vi "TestSquare.vi"(11 "error in (no error)":errorcluster) -> (15 "error out":errorcluster)   [LabVIEW 2016, in "SimpleCalculatorTests.lvlib"]
doc: "Performs square test"
uses:
  SimpleCalculatorTests.lvlib
  APIs/Stimulus/ControlValue/SetValueAuto.vi
  APIs/Get/GetVI/GetVIByName.vi
  APIs/Assert/AssertControlValue/AlmostEqual.vi
  APIs/Stimulus/VI/CloseVI.vi
  Drona.lvlib
  <vilib>/addons/_JKI Toolkits/Caraya/classes/Test/Test.lvclass
  APIs/Stimulus/ControlValue/ControlValue.lvlib
  APIs/Assert/AssertControlValue/AssertControlValue.lvlib
  APIs/Get/GetVI/GetVI.lvlib
  APIs/Stimulus/VI/VI.lvlib
panel:
  # "Drona Test Square"
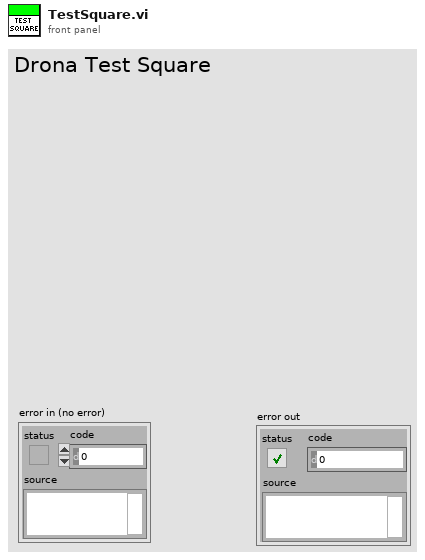
[diagram p1: front panel]
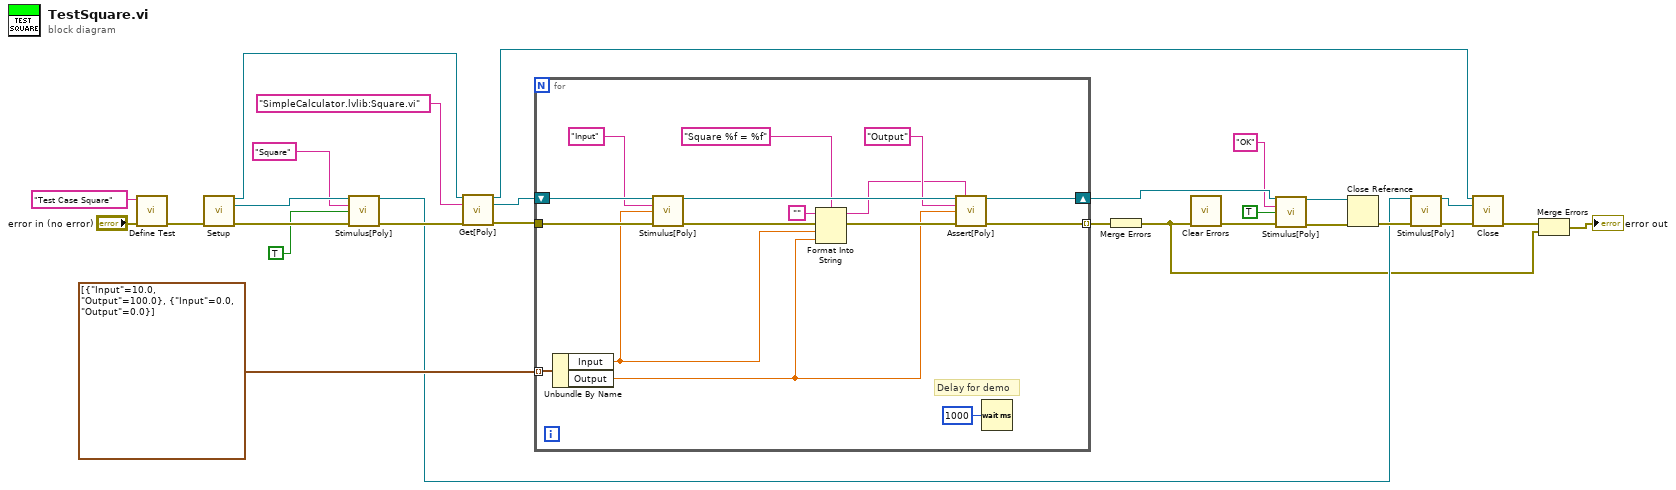
[diagram p0: block diagram]
diagram:
  n1 = call <vilib>:"Define Test.vi"("error in (no error)"="error in (no error)", "Label (VI Title)"="Test Case Square") -> ("error out"=w28:errorcluster)  [unwired: 9 in]
  n2 = call "Setup.vi"("error in"=w28) -> ("Application Ref"=w17:refnum<vi>, "VI Reference Out"=w24:refnum<vi>, "error out"=w25:errorcluster)  [unwired: 12 in]
  n3 = call-poly "Stimulus[Poly].vi"("VI Reference In"=w24, "Control Path"="Square", "Value (Signaling)"=TRUE, "error in"=w25) -> ("VI Reference Out"=w7:refnum<vi>, "error out"=w21:errorcluster)  [unwired: 10 in]
  n4 = call-poly "Get[Poly].vi"("Application Ref in"=w17, "VI Name"="SimpleCalculator.lvlib:Square.vi" ("Control Path"), "error in (no error)"=w21) -> ("Application Ref out"=w16:refnum<vi>, "VI Reference"=w18:refnum<vi>, "error out"=w19:errorcluster)  [unwired: 10 in]
  n5 = for {
    shift-right: [w38] -> w15
    shift-left: w18 -> [w44]
    tunnel: cluster{"Input":dbl, "Output":dbl}[] [{"Input"=10.0, "Output"=100.0}, {"Input"=0.0, "Output"=0.0}] -> [w36] mode=indexing
    tunnel: w19 -> [w43]
    tunnel: [w39] -> w14 mode=indexing
    # "Delay for demo"
    n6 = Unbundle By Name(w36) -> ("Input"=w33:dbl, "Output"=w32:dbl)
    n7 = call-poly "Stimulus[Poly].vi"("VI Reference In"=w44, "Control Path"="Input", "Value (Signaling)"=w33, "error in"=w43) -> ("VI Reference Out"=w40:refnum<vi>, "error out"=w41:errorcluster)  [unwired: 10 in]
    n8 = Format Into String(format string="Square %f = %f", initial string="", error in=w41, w33, w32) -> (resulting string=w31:string, error out=w35:errorcluster)
    n9 = call-poly "Assert[Poly].vi"("VI Reference In"=w40, "Test Label"=w31, "Control Path"="Output", "Control Value"=w32, "Error In"=w35) -> ("VI Reference Out"=w38:refnum<vi>, "Error Out"=w39:errorcluster)  [unwired: 9 in]
    n10 = Wait (ms)(milliseconds to wait=u32 1000) -> ()  [unwired: 1 out]
  }
  n11 = Merge Errors(w14) -> (w2:errorcluster)
  n12 = call <vilib>:"Clear Errors.vi"("error in (no error)"=w2) -> ("error out"=w9:errorcluster)  [unwired: 5 in, 1 out]
  n13 = call-poly "Stimulus[Poly].vi"("VI Reference In"=w15, "Control Path"="OK", "Value (Signaling)"=TRUE, "error in"=w9) -> ("VI Reference Out"=w12:refnum<vi>, "error out"=w13:errorcluster)  [unwired: 10 in]
  n14 = Close Reference(reference=w12, error in (no error)=w13) -> (error out=w8:errorcluster)
  n15 = call-poly "Stimulus[Poly].vi"("VI Reference In"=w7, "error in"=w8) -> ("VI Reference Out"=w6:refnum<vi>, "error out"=w5:errorcluster)  [unwired: 12 in]
  n16 = call "Close.vi"("Application Ref"=w16, "VI Reference"=w6, "error in"=w5) -> ("error out"=w4:errorcluster)  [unwired: 12 in]
  n17 = Merge Errors(w4, w2) -> (→"error out":errorcluster)
